vi "sine xy.vi"() -> ()   [LabVIEW 2012]
panel:
  out "XY Graph":cluster{"Y":dbl[], "Y":dbl[]}[](graph)
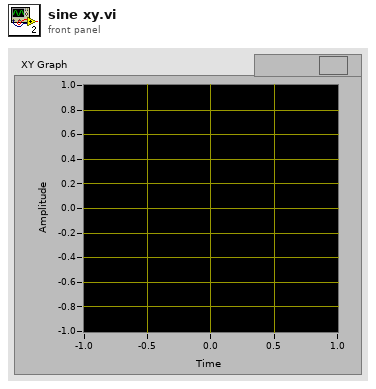
[diagram p1: front panel]
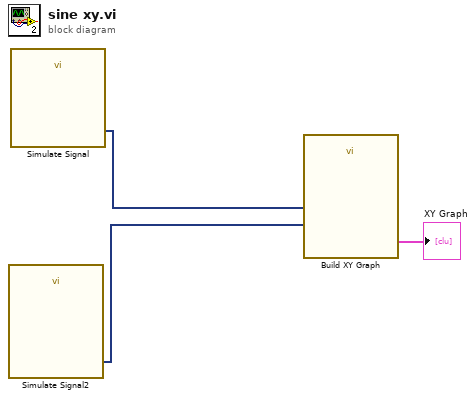
[diagram p0: block diagram]
diagram:
  n1 = call "Simulate Signal2"() -> ("Sine"=w1:dynamicdata)  [unwired: 14 in, 1 out]
  n2 = call "Simulate Signal"() -> ("Sine"=w2:dynamicdata)  [unwired: 14 in, 1 out]
  n3 = call "Build XY Graph"("Y Input"=w1, "X Input"=w2) -> ("XY Graph"=→"XY Graph":cluster{"Y":dbl[], "Y":dbl[]}[])  [unwired: 3 in, 6 out]
